vi "OpenDevice.vi"(4 "RcvLen":u32, 5 "Enable2":bool=TRUE, 6 "DevIndex":u32, 7 "Enable1":bool=TRUE, 8 "error in (no error)":errorcluster caption="错误输入（无错误）", 9 "param":T1[](array[typedef]) {"ACR0" format="%x"}, 10 "Channels":u32[](array[numeric]), 11 "type":u16(ring)=2 items=["USB-CAN"=2, "USB-CAN2.0"=3]) -> (0 "error out":errorcluster caption="错误输出", 3 "open":bool)   [LabVIEW 2011]
uses:
  VIs/Param.ctl
  data/ControlCAN.dll
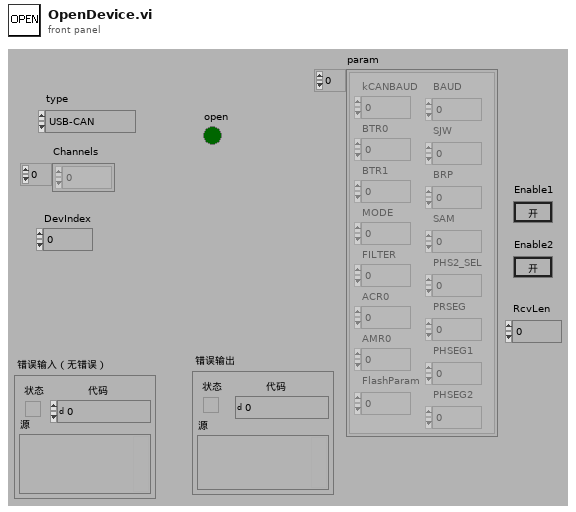
[diagram p1: front panel]
types:
  T1 = typedef "Param.ctl" = cluster{"kCANBAUD":u8, "BTR0":u8, "BTR1":u8, "MODE":u8, "FILTER":u8, "ACR0":u32, "AMR0":u32, "FlashParam":u32, "BAUD":u32, "SJW":u8, "BRP":u8, "SAM":u8, "PHS2_SEL":u8, "PRSEG":u8, "PHSEG1":u8, "PHSEG2":u8}
  T2 = cluster{"AccCode":u32, "AccMask":u32, "Reserved":u32, "Filter":u8, "Timing0":u8, "Timing1":u8, "Mode":u8}
  T3 = enum32{"Bad", "Idle", "Run top level", "Running"}
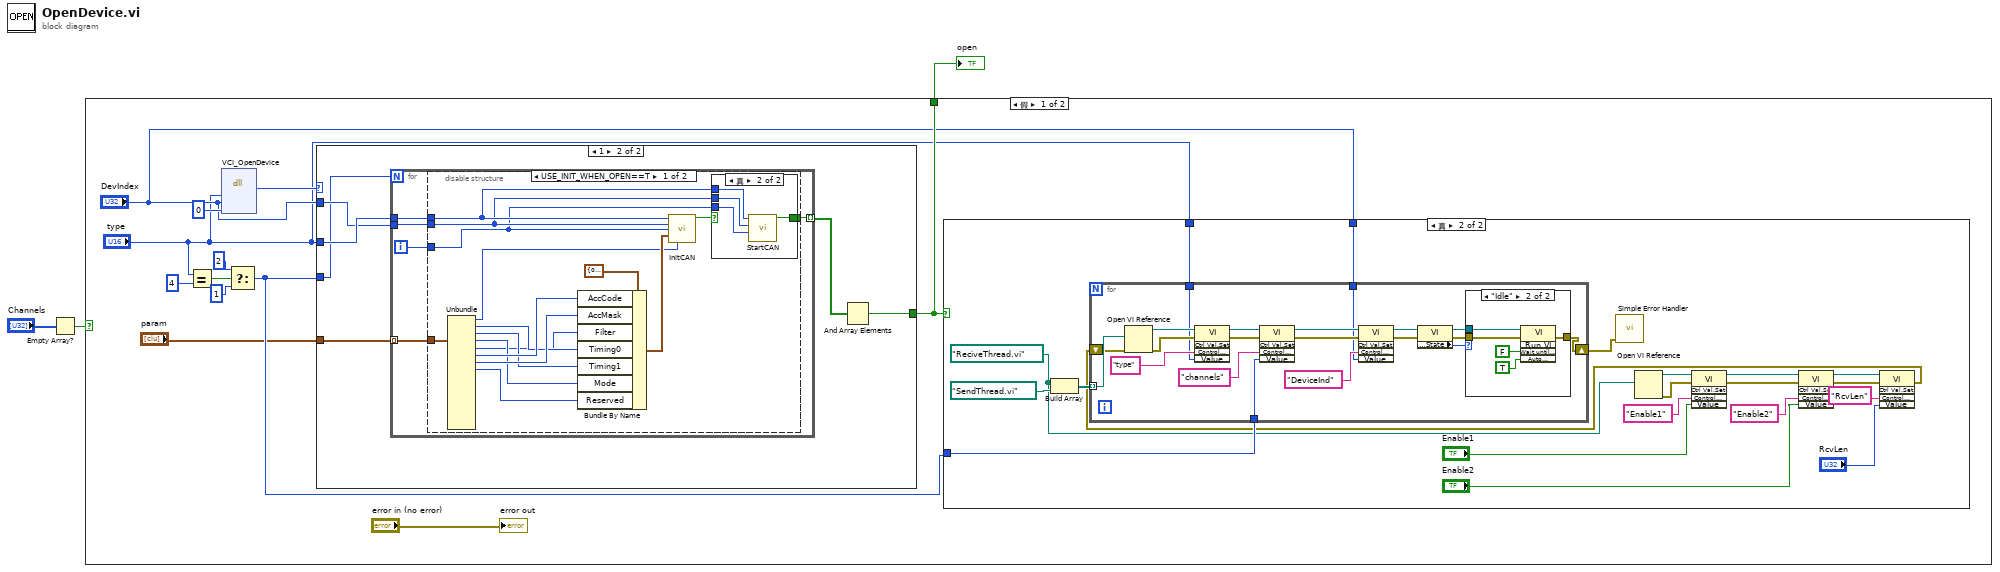
[diagram p0: block diagram]
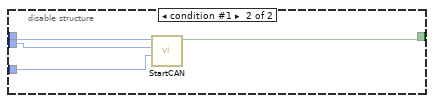
[diagram p6: hidden frame]
diagram:
  n1 = Empty Array?(array="Channels") -> (empty?=w1:bool)
  n2 = case shown="假" w1 {
    tunnel: [w12 _] -> w3
    frame False {
      n3 = Equal?(x="type", y=u16 4) -> (x = y?=w8:bool)
      n4 = dll-call lib="PTH1vabs E工作USB-CAN Tool上位机源码USB-CAN Tool工具源码ZLG版USB CAN TooldataControlCAN.dll" fn="VCI_OpenDevice"("DevType"="type", "DevIndex"="DevIndex", "Reserved"=u32 0 ("DevIndex")) -> ("返回类型"=w15:u32)  [unwired: 6 in, 2 out]
      n5 = Select(t=2 ("y"), s=w8, f=1 ("y")) -> (s? t:f=w5:i32)
      n6 = case shown="1" w15 {
        tunnel: "type" -> [_ w66]
        tunnel: [_ w67] -> w12
        tunnel: "DevIndex" -> [_ w65]
        tunnel: w5 -> [_ w63]
        tunnel: "param" -> [_ w62]
        frame 0, Default {
        }
        frame 1 {
          n7 = for {
            N: w63 -> [_]
            tunnel: w66 -> [w70]
            tunnel: w65 -> [w69]
            tunnel: [w72] -> w64 mode=indexing
            tunnel: w62 -> [w71] mode=indexing
            i -> [w68]
            n8 = disable-structure shown="USE_INIT_WHEN_OPEN==T" {
              disable-tunnel: [w88 w93] -> w72
              disable-tunnel: w71 -> [w87 _]
              disable-tunnel: w70 -> [w79 w96]
              disable-tunnel: w69 -> [w78 w95]
              disable-tunnel: w68 -> [w77 w94]
              frame condition #0 (active) {
                n9 = Unbundle(w87) -> ("kCANBAUD"=w73:u8, "BTR0"=w84:u8, "BTR1"=w83:u8, "MODE"=w82:u8, "FILTER"=w75:u8, "ACR0"=w86:u32, "AMR0"=w85:u32, "FlashParam"=w76:u32)  [unwired: 8 out]
                n10 = Bundle By Name(cluster=T2 {"AccCode"=0, "AccMask"=0, "Reserved"=0, "Filter"=0, "Timing0"=0, "Timing1"=0, "Mode"=0} ("pInitConfig"), "AccCode"=w86, "AccMask"=w85, "Filter"=w75, "Timing0"=w84, "Timing1"=w83, "Mode"=w82, "Reserved"=w76) -> (w81:T2)
                n11 = call "InitCAN.vi"("DeviceType"=w79, "DeviceInd"=w78, "CANInd"=w77, "pInitConfig"=w81, "br"=w73) -> ("Success"=w80:bool)  [unwired: 9 in, 1 out]
                n12 = case shown="真" w80 {
                  tunnel: [_ w92] -> w88
                  tunnel: w79 -> [_ w91]
                  tunnel: w78 -> [_ w90]
                  tunnel: w77 -> [_ w89]
                  frame False {
                  }
                  frame True {
                    n13 = call "StartCAN.vi"("CANInd"=w89, "DeciceInd"=w90, "DeviceType"=w91) -> ("Valid"=w92:bool)  [unwired: 7 in, 1 out]
                  }
                }
              }
              frame condition #1 {
                n14 = call "StartCAN.vi"("CANInd"=w94, "DeciceInd"=w95, "DeviceType"=w96) -> ("Valid"=w93:bool)  [unwired: 7 in, 1 out]
              }
            }
          }
          n15 = And Array Elements(Boolean array=w64) -> (logical AND=w67:bool)
        }
      }
      n16 = case shown="真" w12 {
        tunnel: "type" -> [_ w33]
        tunnel: "DevIndex" -> [_ w32]
        tunnel: w5 -> [_ w31]
        frame False {
        }
        frame True {
          w30 = path "ReciveThread.vi" ("VI路径")
          n17 = Build Array(w30, path "SendThread.vi" ("VI路径")) -> (w35:path[])
          n18 = Open VI Reference(vi path=w30) -> (vi reference=w29:refnum<vi>, error out=w28:errorcluster)  [unwired: 5 in]
          n19 = invoke class="VI" method="Ctrl Val.Set"(reference=w29, error in=w28, "Control Name"="Enable1" ("控件名"), "Value"="Enable1") -> (reference out=w24:refnum<vi>, error out=w23:errorcluster)  [unwired: 1 in, 3 out]
          n20 = invoke class="VI" method="Ctrl Val.Set"(reference=w24, error in=w23, "Control Name"="Enable2" ("控件名"), "Value"="Enable2") -> (reference out=w20:refnum<vi>, error out=w19:errorcluster)  [unwired: 1 in, 3 out]
          n21 = invoke class="VI" method="Ctrl Val.Set"(reference=w20, error in=w19, "Control Name"="RcvLen" ("控件名"), "Value"="RcvLen") -> (error out=w16:errorcluster)  [unwired: 1 in, 4 out]
          n22 = for {
            tunnel: w35 -> [w49] mode=indexing
            tunnel: w33 -> [w45]
            tunnel: w32 -> [w39]
            tunnel: w31 -> [w38]
            shift-right: [w37] -> w21
            shift-left: w16 -> [w36]
            n23 = Open VI Reference(vi path=w49, error in (no error)=w36) -> (vi reference=w55:refnum<vi>, error out=w54:errorcluster)  [unwired: 4 in]
            n24 = invoke class="VI" method="Ctrl Val.Set"(reference=w55, error in=w54, "Control Name"="type" ("控件名"), "Value"=w45) -> (reference out=w52:refnum<vi>, error out=w51:errorcluster)  [unwired: 1 in, 3 out]
            n25 = invoke class="VI" method="Ctrl Val.Set"(reference=w52, error in=w51, "Control Name"="channels" ("控件名"), "Value"=w38) -> (reference out=w42:refnum<vi>, error out=w41:errorcluster)  [unwired: 1 in, 3 out]
            n26 = invoke class="VI" method="Ctrl Val.Set"(reference=w42, error in=w41, "Control Name"="DeviceInd" ("控件名"), "Value"=w39) -> (reference out=w44:refnum<vi>, error out=w43:errorcluster)  [unwired: 1 in, 3 out]
            n27 = property class="VI"(reference=w44, error in=w43) -> (reference out=w47:refnum<vi>, error out=w46:errorcluster, "Exec.State"=w48:T3)
            n28 = case shown="\"Idle\"" w48 {
              tunnel: w47 -> [_ w59]
              tunnel: w46 -> [w56 w58]
              tunnel: [w56 w57] -> w37
              frame "Bad", Default {
              }
              frame "Idle" {
                n29 = invoke class="VI" method="Run VI"(reference=w59, error in=w58, "Wait until done"=FALSE ("结束前等待"), "Auto Dispose Ref"=TRUE ("自动销毁引用")) -> (error out=w57:errorcluster)  [unwired: 1 in, 4 out]
              }
            }
          }
          n30 = call <vilib>:"Simple Error Handler.vi"("error in (no error)"=w21) -> ()  [unwired: 4 in, 5 out]
        }
      }
      "error out" <- "error in (no error)"
    }
    frame True {
    }
  }
  "open" <- w3
